vi "SPC_get_parameter.vi"(6 "SPC Parameter ID":T1 items=["CFD Limit Low", "CFD Limit High", "CFD Zero Cross Level", "CFD Holdoff", "SYNC Zero Cross Level", "SYNC Freq Divider", "SYNC Holdoff", "SYNC Threshold", "TAC Range", "TAC Gain", "TAC Offset", "TAC Limit Low", "TAC Limit High", "ADC Resolution", "External Latch Delay", "Collect Time", "Display Time", "Repeat Time", "Stop On Time", "Stop On Overflow", "Dither Range", "Count Increment", "Memory Bank", "Dead Time Compensation", "Scan Control", "Routing Mode", "TAC Enable Hold", "Operation Mode", "Scan Size X", "Scan Size Y", "Scan Routing X Bits", "Scan Routing Y Bits", "Scan Polarity", "Scan Flyback", "Scan Borders", "Pixel Time", "Pixel Clock Source", "Scan Line Compression", "External Trigger Condition", "External Pixel Clock Divider", "Rate Counting Time", "Macro Time Clock", "ADD Signal Source", "ADC Zoom", "XY Gain", "Image Size X", "Image Size Y", "Image Routing X Bits", "Image Routing Y Bits", "Master Clock", "ADC Sample Delay", "Detector Type", "X Axis Type", "Channel Enable", "Channel Slope", "Channel Spec_no", "TDC_OFFSET1", "TDC_OFFSET2", "TDC_OFFSET3", "TDC_OFFSET4"], 8 "Error In":errorcluster, 10 "Module No":i16 min=0 max=7 step=1, 11 "DLL Path":path) -> (0 "Error Out":errorcluster, 1 "Current Parameter Value":sgl format="%.2f", 2 "Module No":i16, 3 "DLL Path":path)   [LabVIEW 2019]
doc: "The procedure loads ‘value’ with the actual value of the requested parameter from the internal DLL structures of the module ‘mod_no’. The par_id values are defined in spcm_def.h file as SPC_PARAMETERS_KEYWORDS.\nLV users may use the type def /Public/Controls/par_id.ctl\n\ninfo@becker-hickl.com"
uses:
  SPC_Controls/par_id.ctl
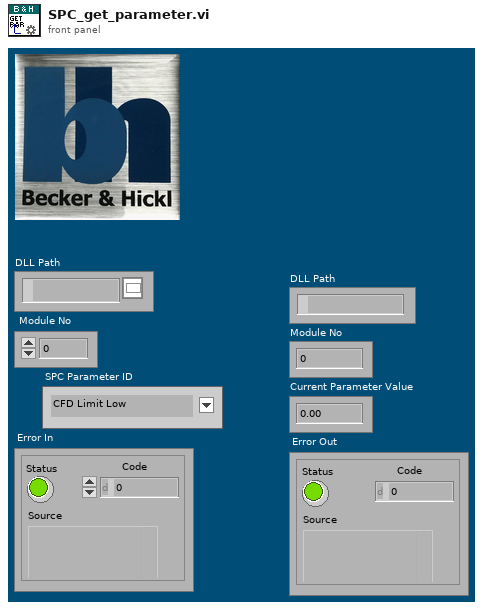
[diagram p1: front panel]
types:
  T1 = typedef "par_id.ctl" = i16
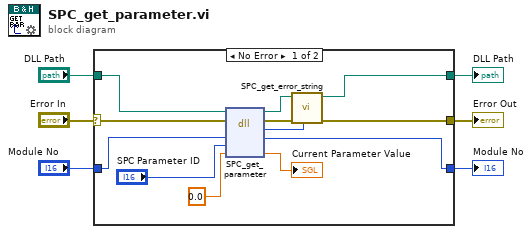
[diagram p0: block diagram]
diagram:
  n1 = case shown="No Error" "Error In" {
    selector: "Error In" -> [w17 w20]
    tunnel: "DLL Path" -> [w18 w21]
    tunnel: [w9 w21] -> w5
    tunnel: [w15 w20] -> w3
    tunnel: "Module No" -> [w14 w19]
    tunnel: [w13 w19] -> w1
    frame No Error {
      n2 = dll-call lib="D:/spcm/lib/lab_view/lv10.0/spcm32.dll" fn="SPC_get_parameter"(path in=w18, error in=w17, "mod_no"=w14, "par_id"="SPC Parameter ID", "value"=sgl 0.0) -> (path out=w10:path, error out=w16:errorcluster, "return type"=w11:i16, "mod_no"=w13:i16, "value"=→"Current Parameter Value":sgl)  [unwired: 2 in]
      n3 = call "SPC_get_error_string.vi"("ErrorID"=w11, "Error In"=w16, "DLL Path"=w10) -> ("Error Out"=w15:errorcluster, "DLL Path"=w9:path)  [unwired: 6 in, 1 out]
    }
    frame Error {
    }
  }
  "Error Out" <- w3
  "DLL Path" <- w5
  "Module No" <- w1
